vi "mosbus.vi"(4 "error in (no error)":errorcluster, 5 "Queue":refnum<queue>, 7 "Event":T1) -> ()   [LabVIEW 2014]
doc: "WhileLoop statemachine Modbus:\n\n- Read Coin, Read Holding va truyen UserEvent neu co su thay doi data.\n- Get cmd tren queue, kiem tra so sanh va thuc hien cmd.\n\n* CMD:\n\n- thay doi ID slaver.\n- Set coin\n- Set Holding.\n- Stop : stop WhileLoop"
uses:
  stateModbus.ctl
  <vilib>/NI/Modbus Library/API/Master/Modbus Master.lvclass
  <vilib>/Platform/TimedLoop/XDataNode/timing_clust.ctl
  <vilib>/Platform/TimedLoop/XDataNode/nitl_modes.ctl
  <vilib>/Platform/TimedLoop/XDataNode/wakeup.ctl
  <vilib>/NI/Modbus Library/API/Modbus API.lvclass/Modbus API.ctl
  <vilib>/NI/Modbus Library/Transmission Data Unit/Transmission Data Unit.lvclass/Transmission Data Unit.ctl
  <vilib>/NI/Modbus Library/Transmission Data Unit/Write Unit ID.vi
  <vilib>/NI/Modbus Library/API/Read Transmission Data Unit.vi
  <vilib>/NI/Modbus Library/API/Write Transmission Data Unit.vi
  <vilib>/NI/Modbus Library/API/Wrapper/Create Serial Master.vi
  <vilib>/platform/TimedLoop/XDataNode/XDataNode.xnode
  <vilib>/Platform/TimedLoop/XDataNode/XDNodeRunTimeDep.lvlib
  <vilib>/NI/Modbus Library/API/Wrapper/API Main.lvlib
  <vilib>/ptbypt/NI_PtbyPt.lvlib
panel:
  out "error out":errorcluster
  out "register values 3":u16[](array[numeric])
  out "coils":bool[](array[boolean])
  in  "ReadHold":T2={"starting address"=0, "number of inputs"=8}
  in  "ReadCoil":T3={"number of inputs"=8, "starting address"=0}
  in  "stop":bool
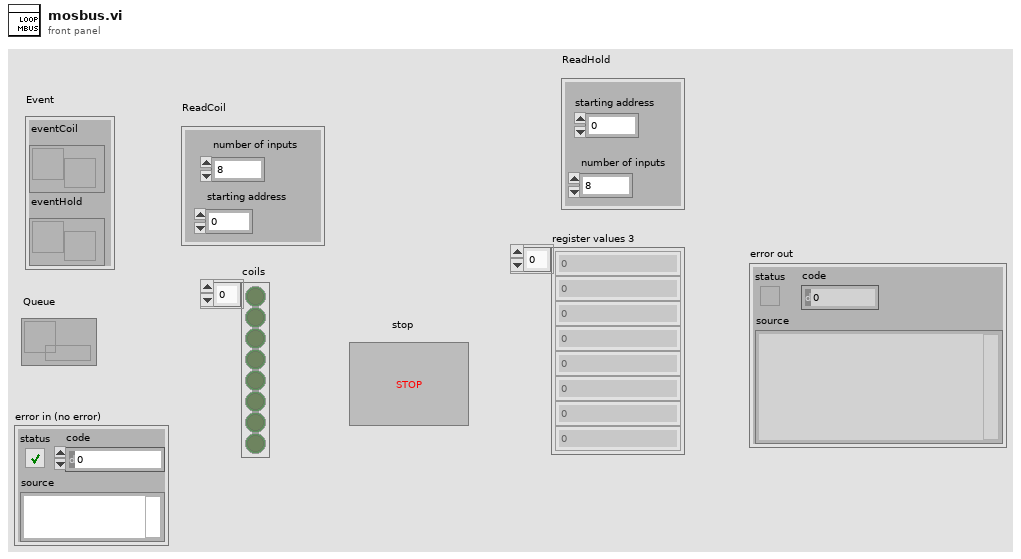
[diagram p1: front panel]
types:
  T1 = cluster{"eventCoil":refnum<user-event>, "eventHold":refnum<user-event>}
  T2 = cluster{"starting address":u16, "number of inputs":u16}
  T3 = cluster{"number of inputs":u16, "starting address":u16}
  T4 = typedef "stateModbus.ctl" = enum16{"Init", "ReadCoin", "ReadHold", "Stop", "Error", "initEventCoil", "initEventHold", "Delay", "CheckQueue"}
  T5 = cluster{"timestamp":u32, "state":T4, "Modbus":refnum<class "Modbus Master.lvclass">, "PollTime":u32, "IDSlaver":u8}
  T6 = typedef "XDNodeRunTimeDep.lvlib/timing_clust.ctl" = cluster{"Expected End [f-1]":u64, "Actual End [f-1]":u64, "Finished Late? [f-1]":bool, "Expected End [i-1]":u64, "Actual End [i-1]":u64, "Finished Late? [i-1]":bool, "Expected Start [i]":u64, "Actual Start [i]":u64, "Expected Start [f]":u64, "Actual Start [f]":u64, "Source Name":string, "Structure Name":string, "Period":i64, "Deadline":i64, "Offset":i64, "Start":i64, "Priority":i32, "Timeout":i32, "Mode":T7, "Wakeup Reason":T8, "Error":errorcluster, "Source Type":string, "Secondary Source Type":string, "Global End Time":u64, "Global Start Time":u64, "Frame Duration":u64, "Iteration Duration":u64, "Assigned CPU":i32, "I/O Scan Engine Mode":u32}
  T7 = typedef "XDNodeRunTimeDep.lvlib/nitl_modes.ctl" = enum32{"No Change", "Process missed periods, maintain original phase", "Discard missed periods, maintain original phase", "Process missed periods, ignore original phase", "Discard missed periods, ignore original phase"}
  T8 = typedef "XDNodeRunTimeDep.lvlib/wakeup.ctl" = enum32{"Normal", "Aborted", "Asynchronous wakeup", "Timing source error", "Timed loop error", "Timeout"}
  T9 = cluster{"StartAddress":u16, "DataHold":u16[], "datacoil":bool, "AddressModbus":u16, "stateCMD":enum16{"WriteCoil", "WriteHold", "ChangeID", "Stop"}}
  T10 = enum16{"WriteCoil", "WriteHold", "ChangeID", "Stop"}
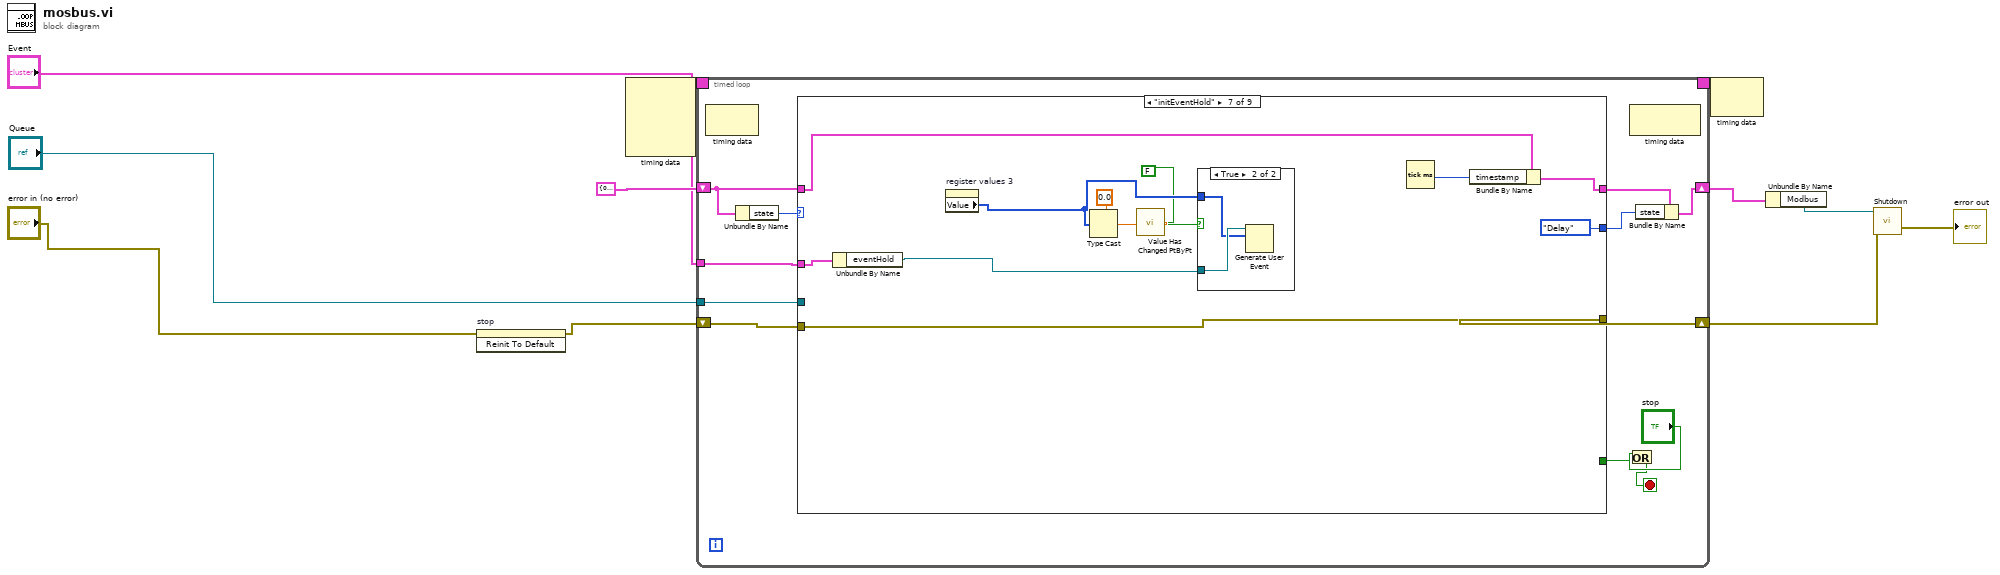
[diagram p0: block diagram]
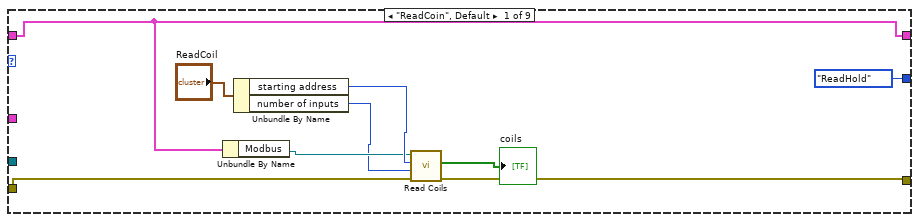
[diagram p2: hidden frame]
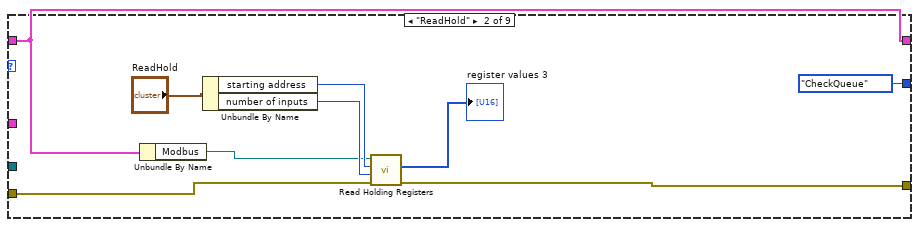
[diagram p3: hidden frame]
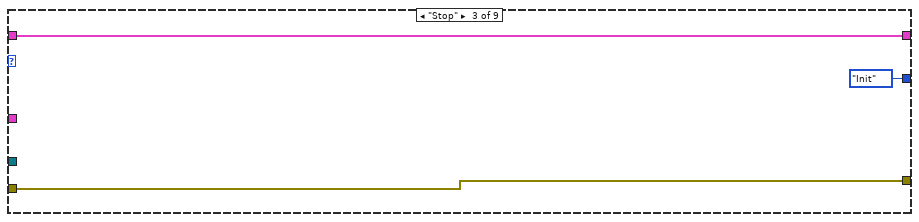
[diagram p4: hidden frame]
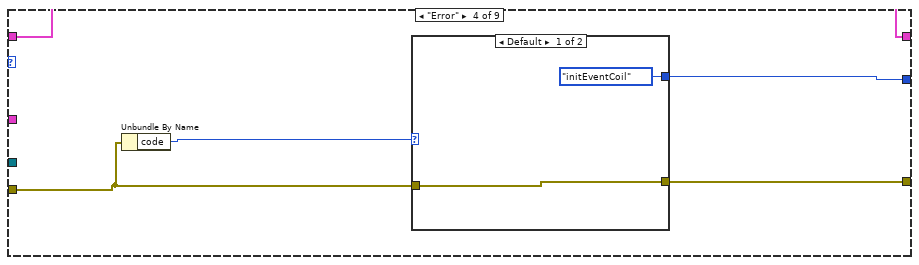
[diagram p5: hidden frame]
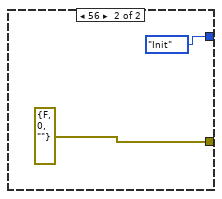
[diagram p6: hidden frame]
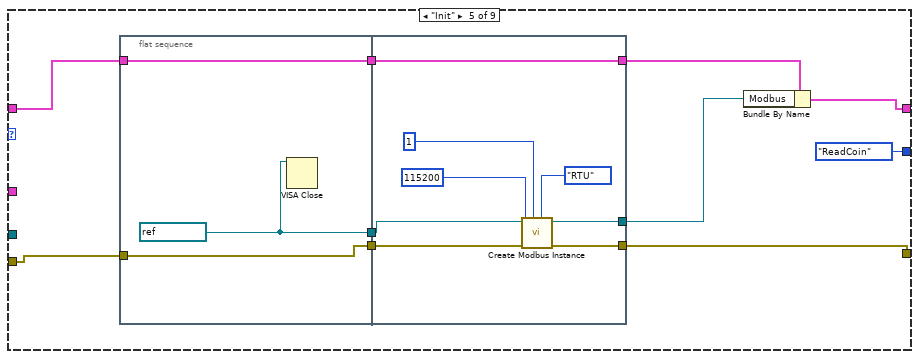
[diagram p7: hidden frame]
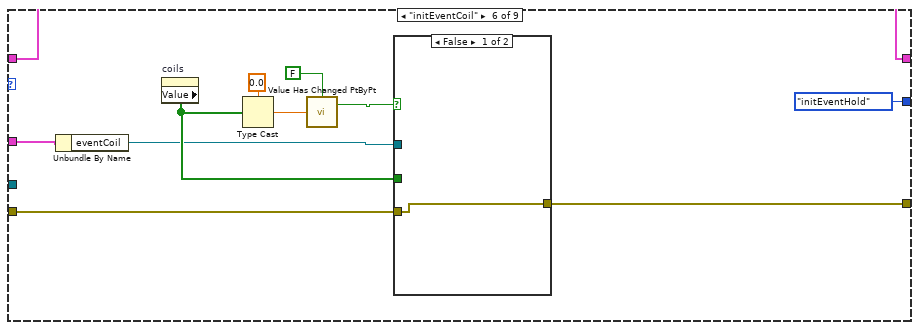
[diagram p8: hidden frame]
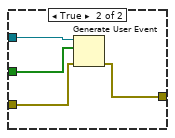
[diagram p9: hidden frame]
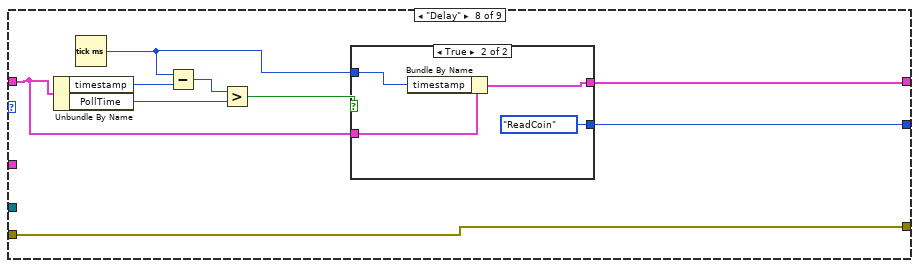
[diagram p11: hidden frame]
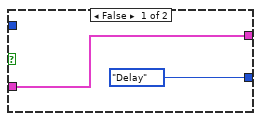
[diagram p12: hidden frame]
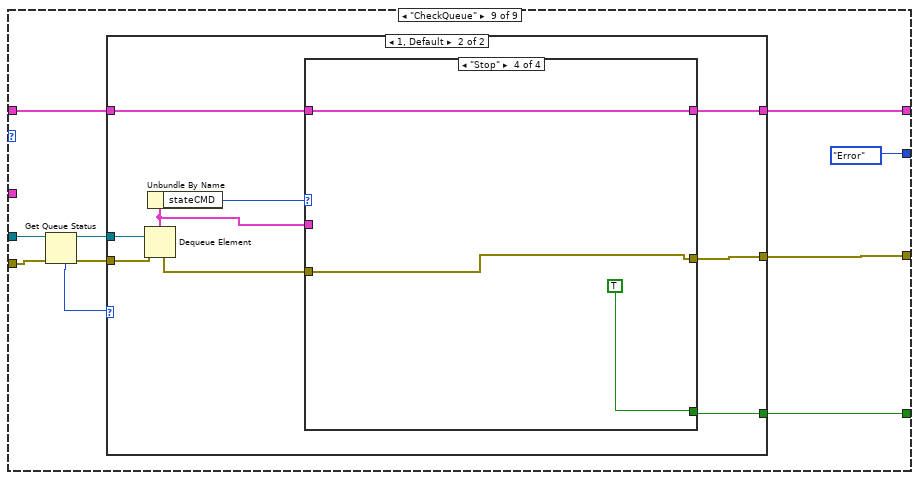
[diagram p13: hidden frame]
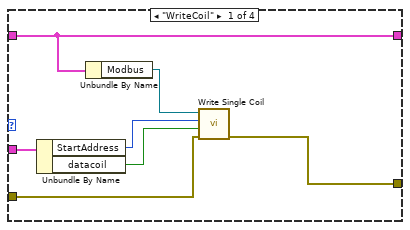
[diagram p15: hidden frame]
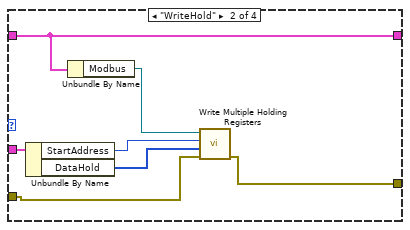
[diagram p16: hidden frame]
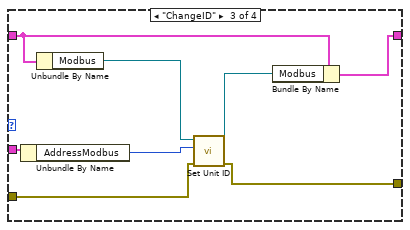
[diagram p17: hidden frame]
diagram:
  n1 = invoke on="stop" class="Bool" method="Reinit To Default"(error in="error in (no error)") -> (error out=w4:errorcluster)  [unwired: 2 in, 2 out]
  n2 = node-c288() -> (w9:T6)  [unwired: 4 in]
  n3 = timed-loop {
    shift-right: [w22] -> w11
    shift-left: w4 -> [w23]
    timing: w9 -> [_]
    timing-out: [_] -> w8
    shift-right: [w17] -> w6
    shift-left: T5 {"timestamp"=0, "state"=enum."Init", "Modbus"=refnum, "PollTime"=100, "IDSlaver"=1} -> [w20]
    tunnel: "Event" -> [w21]
    tunnel: "Queue" -> [w15]
    stop <- w13 stop-if-true
    n4 = node-c288() -> ()  [unwired: 1 in, 1 out]
    n5 = Unbundle By Name(w20) -> ("state"=w19:T4)
    n6 = case shown="\"initEventHold\"" w19 {
      tunnel: w23 -> [w34 w42 w46 w49 w63 w79 w99 w115 w128]
      tunnel: [w33 w43 w46 w50 w64 w78 w99 w115 w126] -> w22
      tunnel: [w28 w36 w44 w47 w60 w80 w96 w112 w122] -> w18
      tunnel: w20 -> [w28 w36 w44 w47 w56 w80 w97 w109 w123]
      tunnel: w21 -> [_ _ _ _ _ w83 w101 _ _]
      tunnel: [stateModbus."ReadHold" ("state") stateModbus."CheckQueue" ("state") stateModbus."Init" ("state") w48 stateModbus."ReadCoin" ("state") stateModbus."initEventHold" ("state") stateModbus."Delay" ("state") w110 stateModbus."Error" ("state")] -> w16
      tunnel: w15 -> [_ _ _ _ _ _ _ _ w131]
      tunnel: [_ _ _ _ _ _ _ _ w125] -> w12
      frame "ReadCoin", Default {
        n7 = Unbundle By Name(w28) -> ("Modbus"=w27:refnum<class "Modbus Master.lvclass">)
        n8 = Unbundle By Name("ReadCoil") -> ("starting address"=w31:u16, "number of inputs"=w26:u16)
        n9 = call-dynamic "Read Coils.vi"("error in"=w34, "number of inputs"=w26, "starting address"=w31, "Modbus master in"=w27) -> ("error out"=w33:errorcluster, "coils"=→"coils":bool[])  [unwired: 5 in, 1 out]
      }
      frame "ReadHold" {
        n10 = Unbundle By Name(w36) -> ("Modbus"=w35:refnum<class "Modbus Master.lvclass">)
        n11 = Unbundle By Name("ReadHold") -> ("starting address"=w41:u16, "number of inputs"=w40:u16)
        n12 = call-dynamic "Read Holding Registers.vi"("error in"=w42, "number of inputs"=w40, "starting address"=w41, "Modbus master in"=w35) -> ("error out"=w43:errorcluster, "register values"=→"register values 3":u16[])  [unwired: 5 in, 1 out]
      }
      frame "Stop" {
      }
      frame "Error" {
        n13 = Unbundle By Name(w49) -> ("code"=w51:i32)
        n14 = case shown="Default" w51 {
          tunnel: [w53 errorcluster {"status"=FALSE, "code"=0, "source"=""} ("error out")] -> w50
          tunnel: w49 -> [w53 _]
          tunnel: [stateModbus."initEventCoil" ("state") stateModbus."Init" ("state")] -> w48
          frame Default {
          }
          frame 56 {
          }
        }
      }
      frame "Init" {
        n15 = flat-sequence {
          tunnel: [w68] -> w65
          tunnel: w63 -> [w67]
          tunnel: [w67] -> w62
          tunnel: [w66] -> w57
          tunnel: w56 -> [w66]
          tunnel: w65 -> [w74]
          tunnel: [w73] -> w59
          tunnel: [w72] -> w64
          tunnel: w62 -> [w71]
          tunnel: [w69] -> w58
          tunnel: w57 -> [w69]
          frame #0 {
            w68 = refnum<visa-resource-name> "USB485" ("VISA resource name")
            n16 = VISA Close(VISA resource name=w68) -> ()  [unwired: 1 in, 1 out]
          }
          frame #1 {
            n17 = call-poly <vilib>:"Create Modbus Instance.vi"("serial type"=enum16{"RTU", "ASCII"}."RTU", "unit ID"=u8 1, "error in"=w71, "baud rate"=u32 115200, "VISA resource name"=w74) -> ("error out"=w72:errorcluster, "serial master instance"=w73:refnum<class "Modbus Master.lvclass">)  [unwired: 5 in]
          }
        }
        n18 = Bundle By Name(cluster=w58, "Modbus"=w59) -> (w60:T5)
      }
      frame "initEventCoil" {
        n19 = Unbundle By Name(w83) -> ("eventCoil"=w82:refnum<user-event>)
        n20 = property on="coils" class="Arr (strict)"() -> ("Value"=w84:bool[])  [unwired: 2 in, 2 out]
        n21 = Type Cast(type=0.0 ("input data point"), x=w84) -> (*(type *) &x=w86:dbl)
        n22 = call <vilib>:"Value Has Changed PtByPt.vi"("input data point"=w86, "initialize"=FALSE) -> ("has changed"=w85:bool)  [unwired: 1 out]
        n23 = case shown="False" w85 {
          tunnel: w84 -> [_ w92]
          tunnel: w82 -> [_ w91]
          tunnel: w79 -> [w88 w90]
          tunnel: [w88 w89] -> w78
          frame False {
          }
          frame True {
            n24 = Generate User Event(user event=w91, event data cluster=w92, error in=w90) -> (error out=w89:errorcluster)  [unwired: 1 in, 1 out]
          }
        }
      }
      frame "initEventHold" {
        n25 = Unbundle By Name(w101) -> ("eventHold"=w100:refnum<user-event>)
        n26 = property on="register values 3" class="Arr (strict)"() -> ("Value"=w94:u16[])  [unwired: 2 in, 2 out]
        n27 = Type Cast(type=0.0 ("input data point"), x=w94) -> (*(type *) &x=w103:dbl)
        n28 = call <vilib>:"Value Has Changed PtByPt.vi"("input data point"=w103, "initialize"=FALSE) -> ("has changed"=w102:bool)  [unwired: 1 out]
        n29 = case shown="True" w102 {
          tunnel: w100 -> [_ w106]
          tunnel: w94 -> [_ w105]
          frame False {
          }
          frame True {
            n30 = Generate User Event(user event=w106, event data cluster=w105) -> ()  [unwired: 2 in, 2 out]
          }
        }
        n31 = Tick Count (ms)() -> (millisecond timer value=w95:u32)
        n32 = Bundle By Name(cluster=w97, "timestamp"=w95) -> (w96:T5)
      }
      frame "Delay" {
        n33 = Unbundle By Name(w109) -> ("timestamp"=w108:u32, "PollTime"=w107:u32)
        n34 = Tick Count (ms)() -> (millisecond timer value=w111:u32)
        n35 = Subtract(x=w111, y=w108) -> (x-y=w114:u32)
        n36 = Greater?(x=w114, y=w107) -> (0:w113:bool)
        n37 = case shown="True" w113 {
          tunnel: [w117 w120] -> w112
          tunnel: w109 -> [w117 w119]
          tunnel: w111 -> [_ w118]
          tunnel: [stateModbus."Delay" ("state") stateModbus."ReadCoin" ("state")] -> w110
          frame False {
          }
          frame True {
            n38 = Bundle By Name(cluster=w119, "timestamp"=w118) -> (w120:T5)
          }
        }
      }
      frame "CheckQueue" {
        n39 = Get Queue Status(queue=w131, error in (no error)=w128) -> (queue out=w129:refnum<queue>, error out=w127:errorcluster, # elements in queue=w130:i32)  [unwired: 1 in, 5 out]
        n40 = case shown="1, Default" w130 {
          tunnel: w129 -> [_ w142]
          tunnel: w127 -> [w133 w140]
          tunnel: [w133 w134] -> w126
          tunnel: [_ w139] -> w125
          tunnel: w123 -> [w132 w137]
          tunnel: [w132 w136] -> w122
          frame 0 {
          }
          frame 1, Default {
            n41 = Dequeue Element(queue=w142, error in (no error)=w140) -> (element=w138:T9, error out=w135:errorcluster)  [unwired: 1 in, 2 out]
            n42 = Unbundle By Name(w138) -> ("stateCMD"=w141:T10)
            n43 = case shown="\"Stop\"" w141 {
              tunnel: [_ _ _ TRUE ("stop")] -> w139
              tunnel: w138 -> [w147 w152 w164 _]
              tunnel: w137 -> [w149 w156 w159 w166]
              tunnel: [w149 w156 w163 w166] -> w136
              tunnel: w135 -> [w144 w153 w158 w165]
              tunnel: [w143 w154 w157 w165] -> w134
              frame "WriteCoil" {
                n44 = Unbundle By Name(w147) -> ("StartAddress"=w146:u16, "datacoil"=w145:bool)
                n45 = Unbundle By Name(w149) -> ("Modbus"=w148:refnum<class "Modbus Master.lvclass">)
                n46 = call-dynamic "Write Single Coil.vi"("error in"=w144, "coil to write"=w145, "address"=w146, "Modbus master in"=w148) -> ("error out"=w143:errorcluster)  [unwired: 6 in, 1 out]
              }
              frame "WriteHold" {
                n47 = Unbundle By Name(w152) -> ("StartAddress"=w151:u16, "DataHold"=w150:u16[])
                n48 = Unbundle By Name(w156) -> ("Modbus"=w155:refnum<class "Modbus Master.lvclass">)
                n49 = call-dynamic "Write Multiple Holding Registers.vi"("error in"=w153, "registers to write"=w150, "starting address"=w151, "Modbus master in"=w155) -> ("error out"=w154:errorcluster)  [unwired: 6 in, 1 out]
              }
              frame "ChangeID" {
                n50 = Unbundle By Name(w164) -> ("AddressModbus"=w160:u16)
                n51 = Unbundle By Name(w159) -> ("Modbus"=w162:refnum<class "Modbus Master.lvclass">)
                n52 = call <vilib>:"Set Unit ID.vi"("error in"=w158, "unit ID"=w160, "Modbus master in"=w162) -> ("error out"=w157:errorcluster, "Modbus master out"=w161:refnum<class "Modbus Master.lvclass">)  [unwired: 7 in]
                n53 = Bundle By Name(cluster=w159, "Modbus"=w161) -> (w163:T5)
              }
              frame "Stop" {
              }
            }
          }
        }
      }
    }
    n54 = Or(x="stop", y=w12) -> (x .or. y?=w13:bool)
    n55 = node-c288() -> ()  [unwired: 1 in, 1 out]
    n56 = Bundle By Name(cluster=w18, "state"=w16) -> (w17:T5)
  }
  n57 = node-c288(w8) -> ()  [unwired: 1 out]
  n58 = Unbundle By Name(w6) -> ("Modbus"=w5:refnum<class "Modbus Master.lvclass">)
  n59 = call-dynamic "Shutdown.vi"("error in"=w11, "Modbus master in"=w5) -> ("error out"=→"error out":errorcluster)  [unwired: 9 in]
